vi "1D Linear Evaluation.vi"(2 "offset":dbl format="%0.2f", 3 "scale":dbl format="%0.2f", 4 "X":dbl[](array[numeric]) format="%0.2f") -> (0 "error":i32, 1 "Y[i]=X[i]*a+b":dbl[](array[numeric]) format="%0.2f")   [LabVIEW 2017, in "NI_AALBase.lvlib"]
doc: "LabVIEW no longer supports this VI. Use the Linear Evaluation VI instead.\nThis VI performs a linear evaluation of the input array <b>X</b>, using <b>scale</b> and <b>offset</b>.\nThis VI calculates the output array <b>Y[i]=X[i]*a+b</b> using the following equation:\nY = aX + b\nwhere a is the multiplicative <b>scale</b> constant and b is the additive constant <b>offset</b>."
uses:
  <vilib>/Analysis/NI_AALBase.lvlib
  <resource>/lvanlys.dll
panel:
  # "Y[i]=X[i]*a+b"
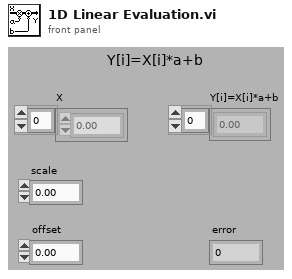
[diagram p1: front panel]
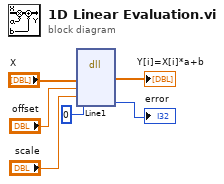
[diagram p0: block diagram]
diagram:
  n1 = dll-call lib="e:/builds/penguin/labview/branches/2017/dev/dist/resource/lvanlys.*" fn="Line1"("X"="X", "offset"="offset", "scale"="scale", 0) -> ("X"=→"Y[i]=X[i]*a+b":dbl[], →"error":i32)  [unwired: 6 in, 2 out]
